vi "Close.vi"(0 "comm interface in":refnum<class "RoboRIO UART.lvclass">, 11 "error in":errorcluster) -> (15 "error out":errorcluster)   [LabVIEW 2018, in "RoboRIO UART.lvclass"]
uses:
  RoboRIO UART.lvclass
  RoboRIO UART.lvclass/RoboRIO UART.ctl
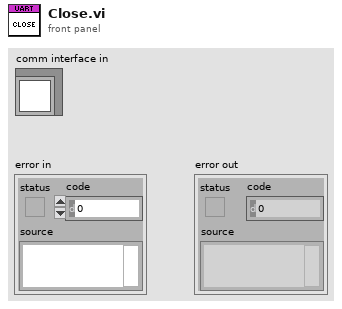
[diagram p1: front panel]
types:
  T1 = typedef "WPI_SerialPortRef.ctl" = cluster{"DevStatus":errorcluster, "Serial Port Name":refnum<visa-resource-name>}
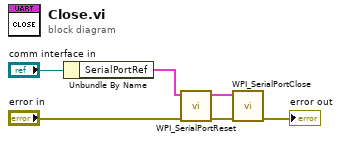
[diagram p0: block diagram]
diagram:
  n1 = Unbundle By Name("comm interface in") -> ("SerialPortRef"=w5:T1)
  n2 = call <vilib>:"WPI_SerialPortReset.vi"("error in (no error)"="error in", "SerialPortRef"=w5) -> ("error out"=w3:errorcluster, "SerialPortRef"=w4:T1)  [unwired: 8 in]
  n3 = call <vilib>:"WPI_SerialPortClose.vi"("error in (no error)"=w3, "SerialPortRef"=w4) -> ("error out"=→"error out":errorcluster)  [unwired: 9 in]
